vi "Cycling_No_DAQ_Tasks_RT.vi"() -> ()   [LabVIEW 2020]
panel:
  in  "Batteryname":string
  out "PS error out":errorcluster
  out "PS Visa Out":refnum<visa-resource-name>
  in  "Battery Type":T1(ring)
  in  "PS type":enum16{"ITECH", "NHR"}(ring)
  in  "PS error in":errorcluster caption="PS error in (no error)"
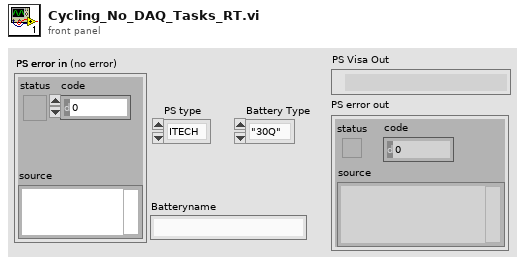
[diagram p1: front panel]
types:
  T1 = enum16{"\"30Q\"", "\"40T\"", "\"2P30Q\"", "\"3P30Q\"", "\"Nissan Leaf\""}
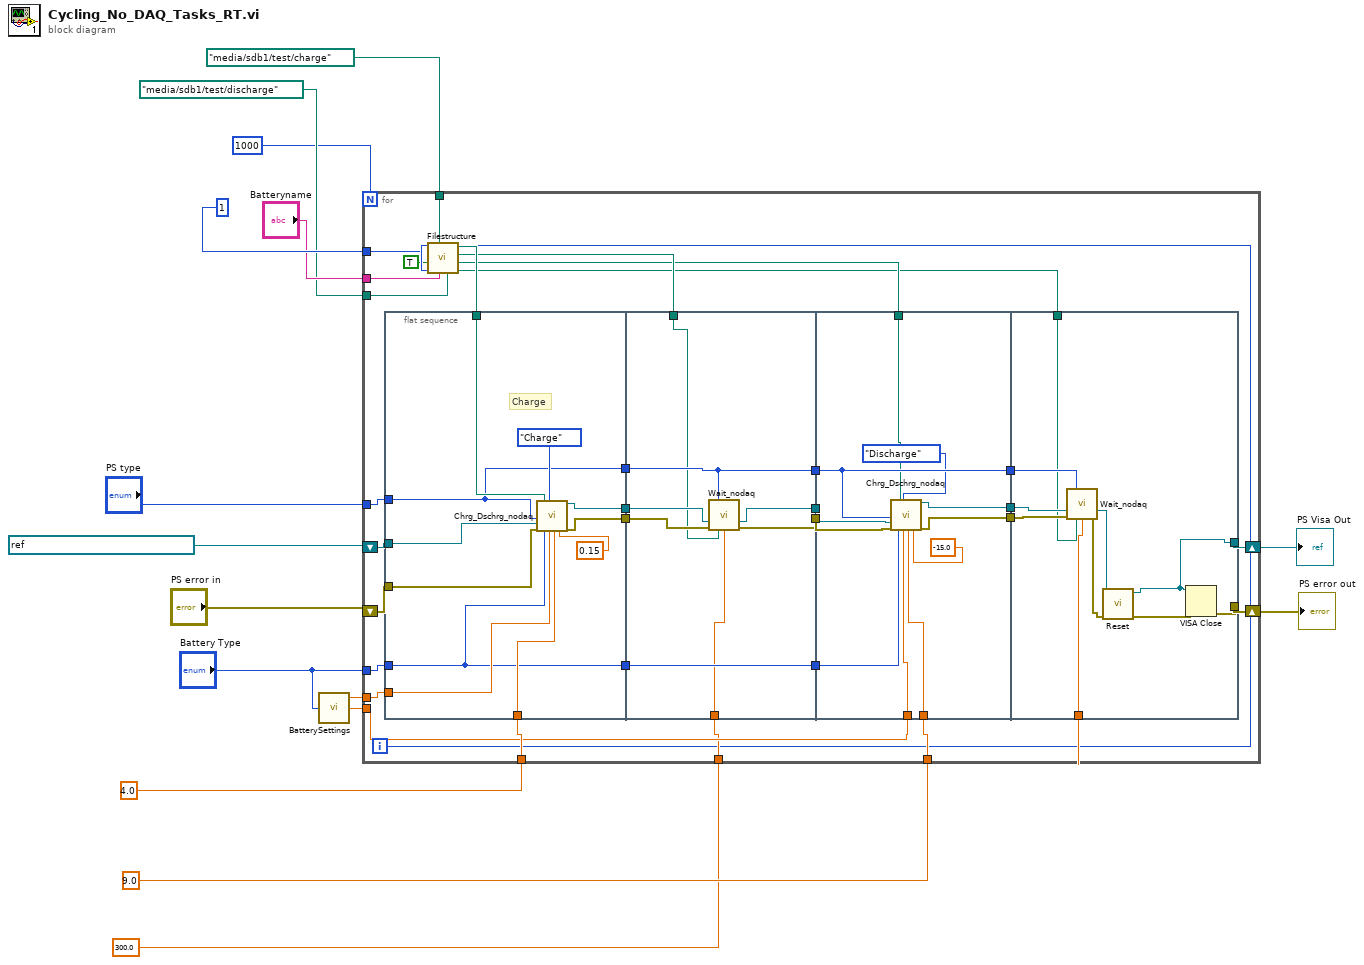
[diagram p0: block diagram]
diagram:
  n1 = call "BatterySettings.vi"("Battery Type"="Battery Type") -> ("Min Voltage (V)"=w10:dbl, "Max Voltage (V)"=w13:dbl)  [unwired: 2 in, 1 out]
  n2 = for {
    N: 1000 ("Number of Cycles") -> [_]
    tunnel: "PS type" -> [w37]
    tunnel: w13 -> [w34]
    tunnel: "Battery Type" -> [w33]
    tunnel: 4.0 ("Charge Current Setpoint") -> [w32]
    tunnel: w10 -> [w31]
    tunnel: 9.0 ("Discharge Current Setpoint") -> [w30]
    tunnel: 300.0 ("Wait time") -> [w25]
    shift-right: [w23] -> w6
    shift-left: refnum<visa-resource-name> "TCPIP0::192.168.0.202::inst0::INSTR" ("PS VISA in") -> [w36]
    shift-right: [w24] -> w7
    shift-left: "PS error in" -> [w35]
    tunnel: 1 ("Starting Cycle") -> [w21]
    tunnel: "Batteryname" -> [w19]
    tunnel: path "/media/sdb1/test/discharge" ("Discharge filepath") -> [w18]
    tunnel: path "/media/sdb1/test/charge" ("Charge filepath") -> [w17]
    i -> [w22]
    n3 = flat-sequence {
      tunnel: w37 -> [w49]
      tunnel: w36 -> [w50]
      tunnel: w35 -> [w51]
      tunnel: w33 -> [w52]
      tunnel: w34 -> [w53]
      tunnel: w32 -> [w54]
      tunnel: [w57] -> w48
      tunnel: [w56] -> w47
      tunnel: [w49] -> w46
      tunnel: [w52] -> w45
      tunnel: w29 -> [w58]
      tunnel: w48 -> [w65]
      tunnel: w47 -> [w64]
      tunnel: w46 -> [w66]
      tunnel: [w60] -> w44
      tunnel: [w61] -> w43
      tunnel: [w66] -> w42
      tunnel: w45 -> [w67]
      tunnel: [w67] -> w41
      tunnel: w28 -> [w63]
      tunnel: w25 -> [w62]
      tunnel: w44 -> [w73]
      tunnel: w43 -> [w74]
      tunnel: w42 -> [w72]
      tunnel: w41 -> [w75]
      tunnel: w31 -> [w76]
      tunnel: w30 -> [w77]
      tunnel: w27 -> [w71]
      tunnel: [w69] -> w40
      tunnel: [w68] -> w39
      tunnel: [w72] -> w38
      tunnel: w26 -> [w81]
      tunnel: w40 -> [w87]
      tunnel: w39 -> [w86]
      tunnel: w25 -> [w82]
      tunnel: w38 -> [w85]
      tunnel: [w88] -> w24
      tunnel: [w80] -> w23
      frame #0 {
        # "Charge"
        n4 = call "Chrg_Dschrg_nodaq.vi"("PS type"=w49, "PS VISA in"=w50, "PS error in"=w51, "CyclePath"=w58, "Battery Type"=w52, "Charge/discharge"=enum8{"Charge", "Discharge"}."Charge", "Charge/Discharge Voltage Setpoint"=w53, "Current Setpoint"=w54, "Current Cutoff"=0.15) -> ("PS VISA out"=w57:refnum<visa-resource-name>, "PS error out"=w56:errorcluster)  [unwired: 9 in]
      }
      frame #1 {
        n5 = call "Wait_nodaq.vi"("PS type"=w66, "PS VISA in"=w65, "PS error in"=w64, "Wait Filepath"=w63, "Wait time"=w62) -> ("PS Visa Out"=w60:refnum<visa-resource-name>, "PS error out"=w61:errorcluster)  [unwired: 9 in]
      }
      frame #2 {
        n6 = call "Chrg_Dschrg_nodaq.vi"("PS type"=w72, "PS VISA in"=w73, "PS error in"=w74, "CyclePath"=w71, "Battery Type"=w75, "Charge/discharge"=enum8{"Charge", "Discharge"}."Discharge", "Charge/Discharge Voltage Setpoint"=w76, "Current Setpoint"=w77, "Current Cutoff"=-15.0) -> ("PS VISA out"=w69:refnum<visa-resource-name>, "PS error out"=w68:errorcluster)  [unwired: 9 in]
      }
      frame #3 {
        n7 = call "Wait_nodaq.vi"("PS type"=w85, "PS VISA in"=w87, "PS error in"=w86, "Wait Filepath"=w81, "Wait time"=w82) -> ("PS Visa Out"=w84:refnum<visa-resource-name>, "PS error out"=w83:errorcluster)  [unwired: 9 in]
        n8 = call "Reset.vi"("error in"=w83, "VISA resource name"=w84) -> ("error out"=w79:errorcluster, "VISA resource name out"=w80:refnum<visa-resource-name>)  [unwired: 8 in]
        n9 = VISA Close(VISA resource name=w80, error in (no error)=w79) -> (error out=w88:errorcluster)
      }
    }
    n10 = call "Filestructure.vi"("Discharge filepath"=w18, "Batteryname"=w19, "Charge filepath"=w17, "For loop i"=w22, "In for loop"=TRUE, "Starting Cycle"=w21) -> ("DischargeWaitPath"=w26:path, "DischargeCyclePath"=w27:path, "ChargeWaitPath"=w28:path, "ChargeCyclePath"=w29:path)  [unwired: 1 in, 1 out]
  }
  "PS error out" <- w7
  "PS Visa Out" <- w6
